vi "Loop_ACT_Telescope.vi"() -> ()   [LabVIEW 2017, in "Arm.lvlib"]
uses:
  Arm.lvlib
  _SHARE ALL/TypeDef Share All/CLUSTER_TalonOutput.ctl
  _SHARE ALL/TypeDef Share All/CLUSTER_TalonInput.ctl
  System Drivers/Phoenix-LabVIEW/Motor Controller/Controls/CTRE_Phoenix_MotorControl_ControlMode.ctl
  TypeDef/CLUSTER_PID.ctl
  _SHARE ALL/TypeDef Share All/CONTROL_PositonGraph.ctl
  Globals/Global_Device_IDs.vi
  _SHARE ALL/Global Share All/Global_STOP.vi
  Global_SM Write_Data Out.vi
  System Drivers/Phoenix-LabVIEW/Motor Controller/Get/CTRE_Phoenix_MotorController_GetSelectedSensorData.vi
  System Drivers/Phoenix-LabVIEW/Motor Controller/Get/CTRE_Phoenix_MotorController_GetVoltage.vi
  Global_ACT Write_Data Out.vi
panel:
  in  "Display Graph":bool
  out "Position Closed Loop Plots":T1
  out "Telescope Input":T2 {"Talon Mode" items=["PercentOutput"=0, "Position"=1, "Velocity"=2, "Current"=3, "Follower"=5, "MotionProfile"=6, "MotionMagic"=7, "MotionMagicArc"=8, "MotionProfileArc"=10, "Disabled"=15]}
  out "Telescope Output":T5
  out "Cycle Time (S)":dbl format="%.3g"
  in  "Target Time(ms)":u32=50
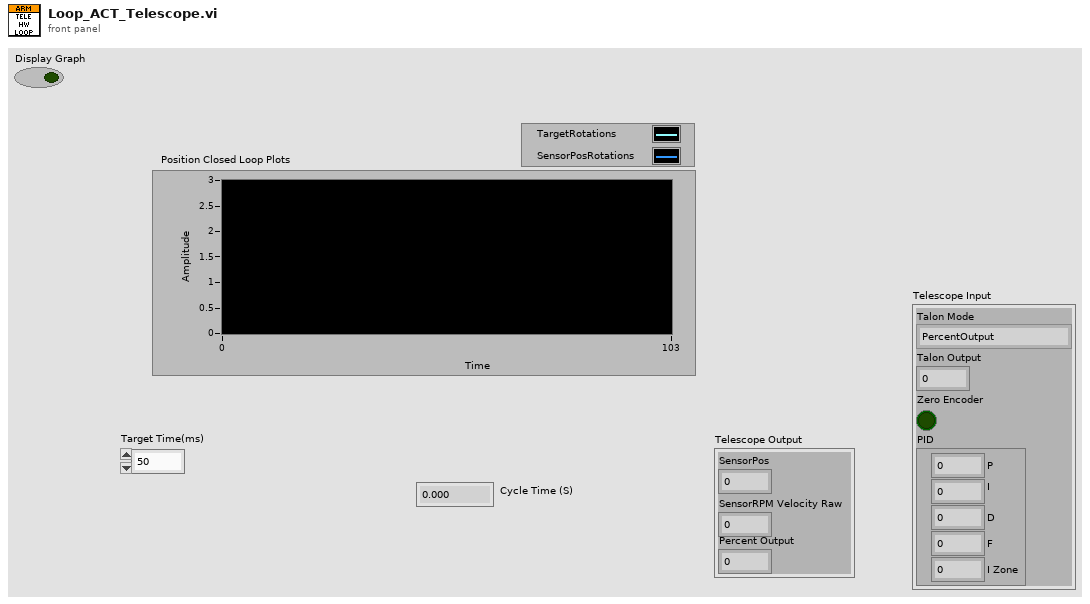
[diagram p1: front panel]
types:
  T1 = typedef "CONTROL_PositonGraph.ctl" = cluster{dbl, "Position (Raw Sensor Units)":i32}
  T2 = typedef "CLUSTER_TalonInput.ctl" = cluster{"Talon Mode":T3, "Talon Output":dbl, "Zero Encoder":bool, "PID":T4}
  T3 = typedef "CTRE_Phoenix_MotorControl_ControlMode.ctl" = u16
  T4 = typedef "CLUSTER_PID.ctl" = cluster{"P":dbl, "I":dbl, "D":dbl, "F":dbl, "I Zone":dbl}
  T5 = typedef "CLUSTER_TalonOutput.ctl" = cluster{"SensorPos":i32, "SensorRPM Velocity Raw":i32, "Percent Output":dbl}
  T6 = typedef "CLUSTER_Arm_Device_IDs.ctl" = cluster{"Elbow Setup":T7, "Telescope Setup":T7, "Elbow Slave Setup":T7, "Telescope Slave Setup":T7}
  T7 = typedef "CLUSTER_Talon_Setup.ctl" = cluster{"Talon SRX ID":u8, "PhaseSensor":bool, "Invert Motor?":bool, "Phoenix Feedback Select":T8, "pidLoopldx":i32, "PID":T4}
  T8 = typedef "CTRE_Phoenix_MotorControl_FeedbackDevice.ctl" = i8
  T9 = typedef "WPI_MotorControlDeviceRef.ctl" = cluster{"DeviceStatus":errorcluster, "Type":T10, "PWM":cluster{"PWM Channel":T11, "DeadBand":T12}, "CAN":cluster{"Device Number":u8, "SetOutput VI Ref":variant, "GetOutput VI Ref":variant, "Enable VI Ref":variant, "Disable VI Ref":variant, "Data":variant}, "Invert":bool, "DIO PWM":cluster{"PWM \"Enable\" Channel":T11, "DIOChannel":T13, "PWM Rate":dbl}}
  T10 = typedef "WPI_MotorControlType.ctl" = enum16{"PWM", "CAN", "DIO PWM"}
  T11 = typedef "FPGA_DIOPWMChannel.ctl" = enum8{"PWM 0", "PWM 1", "PWM 2", "PWM 3", "PWM 4", "PWM 5", "PWM 6", "PWM 7", "PWM 8", "PWM 9", "PWM MXP 0", "PWM MXP 1", "PWM MXP 2", "PWM MXP 3", "PWM MXP 4", "PWM MXP 5", "PWM MXP 6", "PWM MXP 7", "PWM MXP 8", "PWM MXP 9", "Invalid"}
  T12 = typedef "WPI_PWMDeadband.ctl" = cluster{"Name":string, "maxPositivePwm":i32, "minPositivePwm":i32, "centerPwm":i32, "maxNegativePwm":i32, "minNegativePwm":i32, "angularRange":u16}
  T13 = typedef "FPGA_DIOChannel.ctl" = enum8{"DIO 0", "DIO 1", "DIO 2", "DIO 3", "DIO 4", "DIO 5", "DIO 6", "DIO 7", "DIO 8", "DIO 9", "DIO MXP 0", "DIO MXP 1", "DIO MXP 2", "DIO MXP 3", "DIO MXP 4", "DIO MXP 5", "DIO MXP 6", "DIO MXP 7", "DIO MXP 8", "DIO MXP 9", "DIO MXP 10", "DIO MXP 11", "DIO MXP 12", "DIO MXP 13", "DIO MXP 14", "DIO MXP 15", "SPI Port CS1", "SPI Port CS2", "SPI Port CS3", "SPI Port MISO", "SPI Port MOSI", "Invalid"}
  T14 = cluster{"PhoenixMotorControlDevRef":T9, "Telescope Output":T5, "Telescope Input":T2, "Target Time(ms)":u32, "Current Time":timestamp, "Previous Time":timestamp, "Cycle Time (S)":dbl, "Last PID":T4}
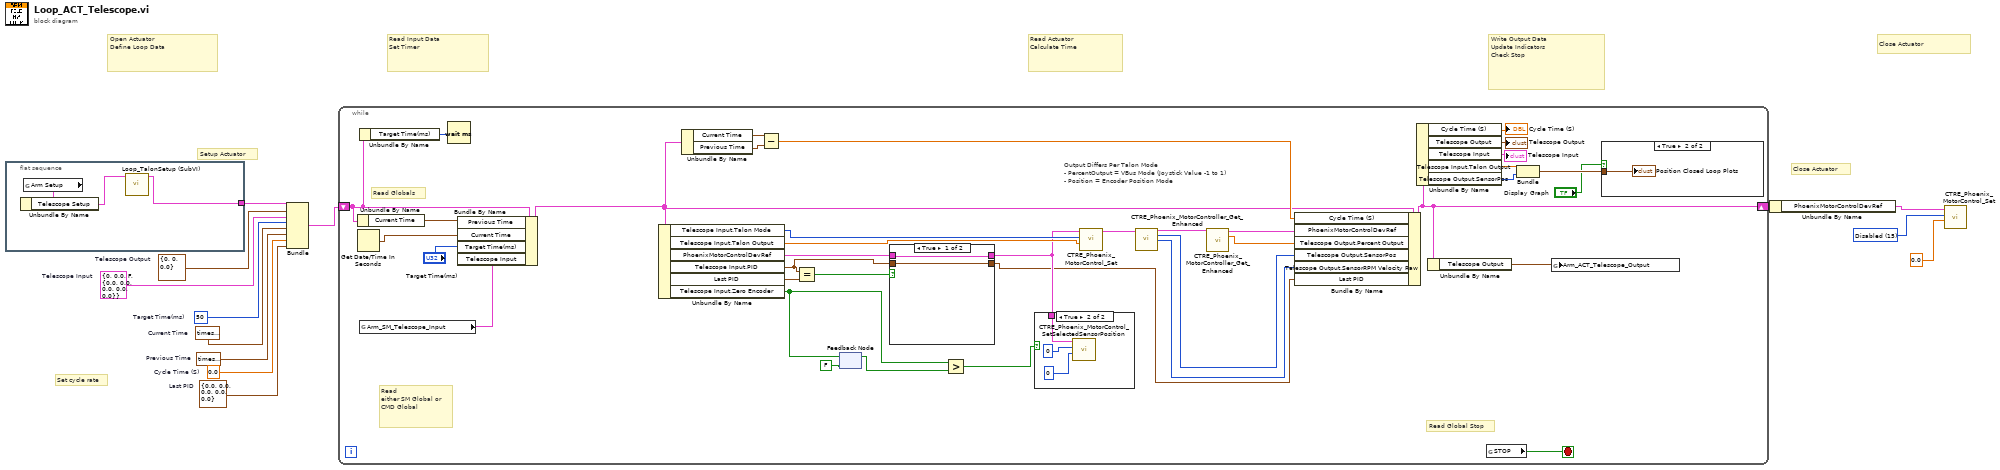
[diagram p0: block diagram]
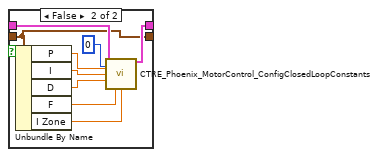
[diagram p2: hidden frame]
diagram:
  w1 = T4 {"P"=0.0, "I"=0.0, "D"=0.0, "F"=0.0, "I Zone"=0.0}  # Last PID
  w3 = T3 15 items=["PercentOutput"=0, "Position"=1, "Velocity"=2, "Current"=3, "Follower"=5, "MotionProfile"=6, "MotionMagic"=7, "MotionMagicArc"=8, "MotionProfileArc"=10, "Disabled"=15] ("Control Mode")
  w5 = T5 {"SensorPos"=0, "SensorRPM Velocity Raw"=0, "Percent Output"=0.0}  # Telescope Output
  w6 = T2 {"Talon Mode"=0, "Talon Output"=0.0, "Zero Encoder"=FALSE, "PID"={"P"=0.0, "I"=0.0, "D"=0.0, "F"=0.0, "I Zone"=0.0}}  # Telescope Input
  w8 = 0.0  # Cycle Time (S)
  w13 = timestamp(0 s since 1904-01-01)  # Previous Time
  w12 = timestamp(0 s since 1904-01-01)  # Current Time
  w11 = u32 50  # Target Time(ms)
  # "Close Actuator"
  # "Write Output Data\nUpdate Indicators\nCheck Stop"
  # "Read Actuator\nCalculate Time"
  # "Read Input Data\nSet Timer"
  # "Open Actuator\nDefine Loop Data"
  # "Set cycle rate"
  # "Close Actuator"
  # "Setup Actuator"
  n1 = flat-sequence {
    tunnel: [w14] -> w7
    frame #0 {
      n2 = global read "Global_Device_IDs.vi" "Arm Setup"() -> (w16:T6)
      n3 = Unbundle By Name(w16) -> ("Telescope Setup"=w15:T7)
      n4 = call "Loop_TalonSetup (SubVI).vi"("Elbow Setup"=w15) -> ("PhoenixMotorControlDevRef"=w14:T9)  [unwired: 10 in]
    }
  }
  n5 = Bundle("PhoenixMotorControlDevRef"=w7, "Telescope Output"=w5, "Telescope Input"=w6, "Target Time(ms)"=w11, "Current Time"=w12, "Previous Time"=w13, "Cycle Time (S)"=w8, "Last PID"=w1) -> (w10:T14)  [unwired: 1 in]
  n6 = while {
    shift-right: [w46] -> w9
    shift-left: w10 -> [w48]
    stop <- w54 stop-if-true
    # "Output Differs Per Talon Mode\n- PercentOutput = VBus Mode (Joystick Value -1 to 1)\n- Position = Encoder Position Mode"
    # "Read\neither SM Global or CMD Global"
    # "Read Globals"
    # "Read Global Stop"
    n7 = Unbundle By Name(w48) -> ("Current Time"=w52:timestamp)
    n8 = Get Date/Time In Seconds() -> (seconds since 1Jan1904=w53:timestamp)
    n9 = Unbundle By Name(w48) -> ("Target Time(ms)"=w47:u32)
    n10 = global read "Global_SM Write_Data Out.vi" "Arm_SM_Telescope_Input"() -> (w42:T2)
    n11 = Wait (ms)(milliseconds to wait=w47) -> ()  [unwired: 1 out]
    n12 = Bundle By Name(cluster=w48, "Previous Time"=w52, "Current Time"=w53, "Target Time(ms)"="Target Time(ms)", "Telescope Input"=w42) -> (w28:T14)
    n13 = Unbundle By Name(w28) -> ("Telescope Input.Talon Mode"=w41:T3, "Telescope Input.Talon Output"=w40:dbl, "PhoenixMotorControlDevRef"=w27:T9, "Telescope Input.PID"=w23:T4, "Last PID"=w24:T4, "Telescope Input.Zero Encoder"=w18:bool)
    n14 = Unbundle By Name(w28) -> ("Current Time"=w51:timestamp, "Previous Time"=w50:timestamp)
    n15 = Subtract(x=w51, y=w50) -> (x-y=w44:dbl)
    n16 = Equal?(x=w23, y=w24) -> (x = y?=w21:bool)
    n17 = feedback #1(FALSE) -> (w19:bool)
    n18 = feedback-in #1(w18) -> ()
    n19 = case shown="True" w21 {
      tunnel: w27 -> [w56 w65]
      tunnel: [w56 w64] -> w26
      tunnel: w23 -> [w55 w57]
      tunnel: [w55 w57] -> w22
      frame True {
      }
      frame False {
        n20 = Unbundle By Name(w57) -> ("P"=w62:dbl, "I"=w61:dbl, "D"=w60:dbl, "F"=w59:dbl, "I Zone"=w58:dbl)
        n21 = call "CTRE_Phoenix_MotorControl_ConfigClosedLoopConstants.vi"("PhoenixMotorControlDevRef"=w65, "slotIdx"=0, "P"=w62, "I"=w61, "D"=w60, "F"=w59, "I Zone"=w58) -> ("PhoenixMotorControlDevRef"=w64:T9)  [unwired: 7 in, 1 out]
      }
    }
    n22 = Greater?(x=w18, y=w19) -> (0:w17:bool)
    n23 = case shown="True" w17 {
      tunnel: w26 -> [_ w69]
      frame False {
      }
      frame True {
        n24 = call "CTRE_Phoenix_MotorControl_SetSelectedSensorPosition.vi"("pidLoopIdx"=u32 0, "New Sensor Position"=0, "PhoenixMotorControlDevRef"=w69) -> ()  [unwired: 7 in, 2 out]
      }
    }
    n25 = call "CTRE_Phoenix_MotorControl_Set.vi"("Output"=w40, "Control Mode"=w41, "PhoenixMotorControlDevRef"=w26) -> ("PhoenixMotorControlDevRef"=w39:T9)  [unwired: 7 in, 1 out]
    n26 = call-poly "CTRE_Phoenix_MotorController_Get_Enhanced.vi"("PhoenixMotorControlDevRef"=w39) -> ("PhoenixMotorControlDevRef"=w38:T9, "Position (Raw Sensor Units)"=w34:i32, "Velocity (Raw Sensor Units per 100 ms)"=w35:i32)  [unwired: 11 in, 1 out]
    n27 = call-poly "CTRE_Phoenix_MotorController_Get_Enhanced.vi"("PhoenixMotorControlDevRef"=w38) -> ("PhoenixMotorControlDevRef"=w37:T9, "Percent Output"=w36:dbl)  [unwired: 10 in, 3 out]
    n28 = Bundle By Name(cluster=w28, "Cycle Time (S)"=w44, "PhoenixMotorControlDevRef"=w37, "Telescope Output.Percent Output"=w36, "Telescope Output.SensorPos"=w34, "Telescope Output.SensorRPM Velocity Raw"=w35, "Last PID"=w22) -> (w46:T14)
    n29 = Unbundle By Name(w46) -> ("Cycle Time (S)"=→"Cycle Time (S)":dbl, "Telescope Output"=→"Telescope Output":T5, "Telescope Input"=→"Telescope Input":T2, "Telescope Input.Talon Output"=w31:dbl, "Telescope Output.SensorPos"=w30:i32)
    n30 = Unbundle By Name(w46) -> ("Telescope Output"=w43:T5)
    n31 = global read "Global_STOP.vi" "STOP"() -> (w54:bool)
    n32 = Bundle("Talon Output"=w31, "SensorPos"=w30) -> (w29:cluster{"Talon Output":dbl, "SensorPos":i32})  [unwired: 1 in]
    n33 = global write "Global_ACT Write_Data Out.vi" "Arm_ACT_Telescope_Output"(w43) -> ()
    n34 = case shown="True" "Display Graph" {
      tunnel: w29 -> [_ w66]
      frame False {
      }
      frame True {
        "Position Closed Loop Plots" <- w66
      }
    }
  }
  n35 = Unbundle By Name(w9) -> ("PhoenixMotorControlDevRef"=w4:T9)
  n36 = call "CTRE_Phoenix_MotorControl_Set.vi"("Output"=0.0, "Control Mode"=w3, "PhoenixMotorControlDevRef"=w4) -> ()  [unwired: 7 in, 2 out]
